vi "FR GUI DC meter setup.vi"(11 "DC meter":T2={"DC meter type"=enum."H/A/K 3458", "DC meter VISA"="", "NPLC"=10, "status ref"=refnum}) -> (3 "DC meter out":T2={"DC meter type"=enum."H/A/K 3458", "DC meter VISA"="", "NPLC"=10, "status ref"=refnum})   [LabVIEW 2020]
doc: "Use this template to build a producer/consumer design pattern with events to produce queue items. Use this design pattern instead of the User Interface Event Handler pattern for user interfaces when you want to execute code asynchronously in response to an event without slowing the user interface responsiveness."
uses:
  General DC meter/Type definitions/DC meter.ctl
  General DC meter/Type definitions/DC meter type.ctl
  <vilib>/Utility/error.llb/DialogType.ctl
  <vilib>/Utility/error.llb/Error Cluster From Error Code.vi
  <vilib>/ErrorRing/Error Ring.xnode
  external libraries/varilib/varilib.lvlib
panel:
  out "not tested label":string="This device is not\nyet fully tested!"
  in  "NPLC":i32=10 min=1
  in  "DC meter type":T1
  in  "VISA":refnum<visa-resource-name>
  out "gui_elements":refnum<vi>[](array[refnum])
  out "Status":string
  in  "save_and_quit":bool
  in  "test":bool
  in  "cancel":bool
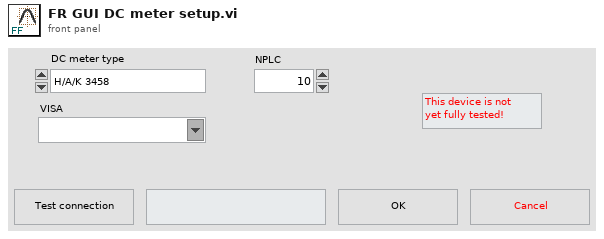
[diagram p1: front panel]
types:
  T1 = typedef "DC meter type.ctl" = enum16{"H/A/K 3458", "FLuke 8508A", "dummy"}
  T2 = typedef "DC meter.ctl" = cluster{"DC meter type":T1, "DC meter VISA":refnum<visa-resource-name>, "NPLC":i32, "status ref":refnum<vi>}
  T3 = typedef "DialogType.ctl" = u16
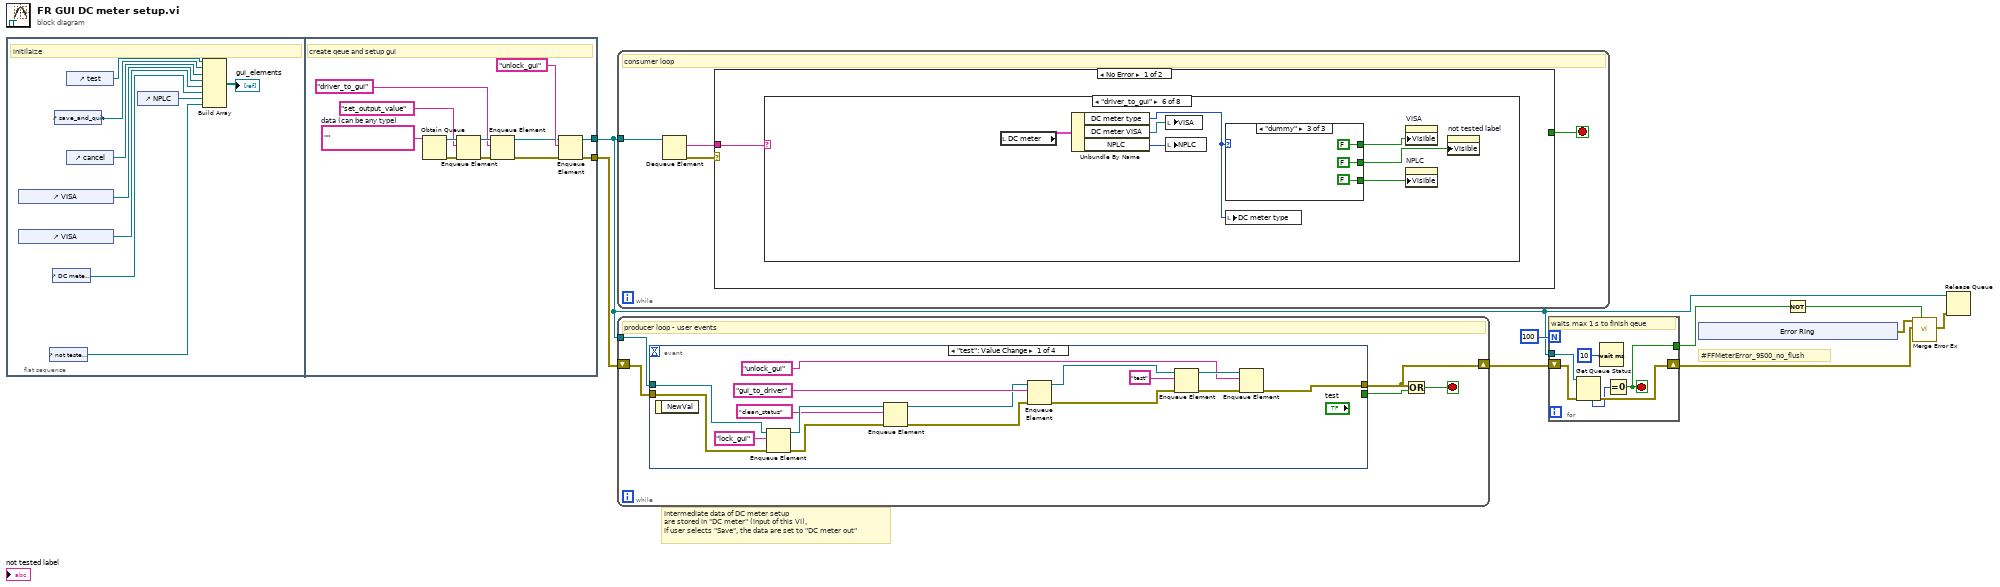
[diagram p0: block diagram]
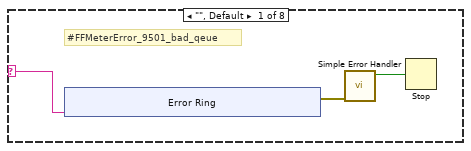
[diagram p2: hidden frame]
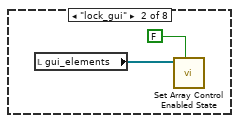
[diagram p3: hidden frame]
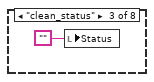
[diagram p4: hidden frame]
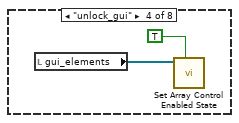
[diagram p5: hidden frame]
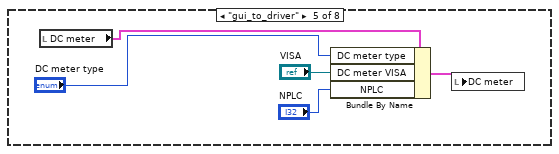
[diagram p6: hidden frame]
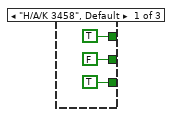
[diagram p7: hidden frame]
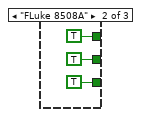
[diagram p8: hidden frame]
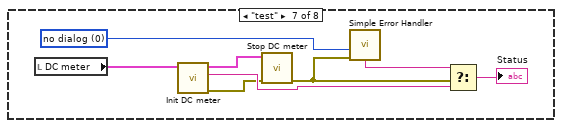
[diagram p9: hidden frame]
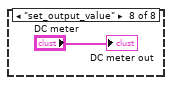
[diagram p10: hidden frame]
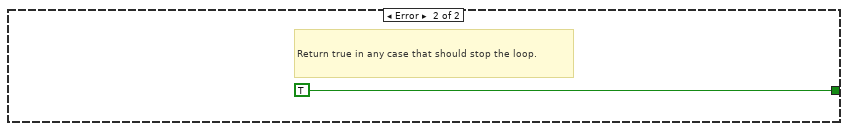
[diagram p11: hidden frame]
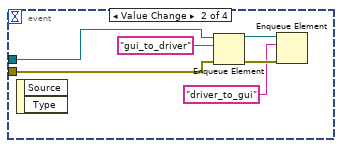
[diagram p12: hidden frame]
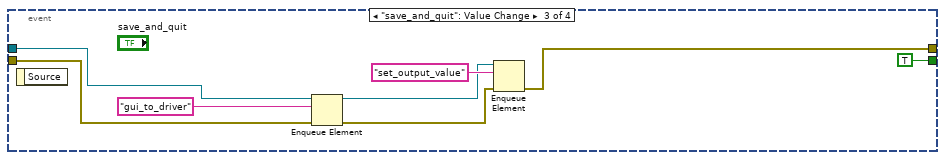
[diagram p13: hidden frame]
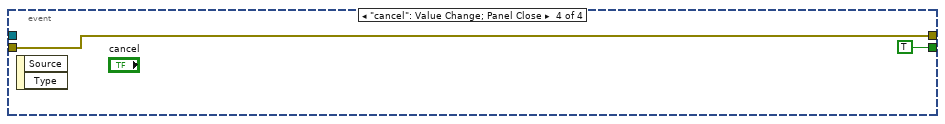
[diagram p14: hidden frame]
diagram:
  # "#FFMeterError_9500_no_flush"
  # "intermediate data of DC meter setup\nare stored in \"DC meter\" (input of this VI),\nif user selects \"Save\", the data are set to \"DC meter out\""
  n1 = flat-sequence {
    tunnel: [w23] -> w2
    tunnel: [w21] -> w1
    frame #0 {
      # "initilaize"
      n2 = control-ref of="VISA"() -> (w12:refnum<vi>)
      n3 = control-ref of="VISA"() -> (w14:refnum<vi>)
      n4 = control-ref of="not tested label"() -> (w10:refnum<vi>)
      n5 = control-ref of="DC meter type"() -> (w13:refnum<vi>)
      n6 = control-ref of="save_and_quit"() -> (w17:refnum<vi>)
      n7 = control-ref of="test"() -> (w18:refnum<vi>)
      n8 = control-ref of="cancel"() -> (w16:refnum<vi>)
      n9 = control-ref of="NPLC"() -> (w11:refnum<vi>)
      n10 = Build Array(w18, w17, w16, w12, w14, w13, w11, w10) -> (→"gui_elements":refnum<vi>[])
    }
    frame #1 {
      w22 = ""  # data (can be any type)
      # "create qeue and setup gui"
      n11 = Obtain Queue(element data type=w22) -> (queue out=w27:refnum<queue>, error out=w29:errorcluster)  [unwired: 4 in, 1 out]
      n12 = Enqueue Element(queue=w27, element="set_output_value", error in (no error)=w29) -> (queue out=w28:refnum<queue>, error out=w30:errorcluster)  [unwired: 1 in, 1 out]
      n13 = Enqueue Element(queue=w28, element="driver_to_gui", error in (no error)=w30) -> (queue out=w19:refnum<queue>, error out=w20:errorcluster)  [unwired: 1 in, 1 out]
      n14 = Enqueue Element(queue=w19, element="unlock_gui", error in (no error)=w20) -> (queue out=w23:refnum<queue>, error out=w21:errorcluster)  [unwired: 1 in, 1 out]
    }
  }
  n15 = while {
    tunnel: w2 -> [w34]
    stop <- w31 stop-if-true
    # "consumer loop"
    n16 = Dequeue Element(queue=w34) -> (element=w32:string, error out=w33:errorcluster)  [unwired: 2 in, 2 out]
    n17 = case shown="No Error" w33 {
      tunnel: w32 -> [w35 _]
      tunnel: [_ TRUE] -> w31
      frame No Error {
        n18 = case shown="\"driver_to_gui\"" w35 {
          selector: w35 -> [w36 _ _ _ _ _ _ _]
          frame "", Default {
            # "#FFMeterError_9501_bad_qeue"
            n19 = xnode "Error Ring"("parameter 0"=w36) -> ("error out"=w38:errorcluster)
            n20 = call <vilib>:"Simple Error Handler.vi"("error in (no error)"=w38) -> ("error?"=w37:bool)  [unwired: 4 in, 4 out]
            n21 = Stop(stop? (T)=w37) -> ()
          }
          frame "lock_gui" {
            n22 = local read "gui_elements"() -> (w47:refnum<vi>[])
            n23 = call "Set Array Control Enabled State.vi"("enabled (T)"=FALSE, "reference array in"=w47) -> ()  [unwired: 8 in, 2 out]
          }
          frame "clean_status" {
            n24 = local write "Status"("") -> ()
          }
          frame "unlock_gui" {
            n25 = local read "gui_elements"() -> (w50:refnum<vi>[])
            n26 = call "Set Array Control Enabled State.vi"("enabled (T)"=TRUE, "reference array in"=w50) -> ()  [unwired: 8 in, 2 out]
          }
          frame "gui_to_driver" {
            n27 = local read "DC meter"() -> (w54:T2)
            n28 = Bundle By Name(cluster=w54, "DC meter type"="DC meter type", "DC meter VISA"="VISA", "NPLC"="NPLC") -> (w55:T2)
            n29 = local write "DC meter"(w55) -> ()
          }
          frame "driver_to_gui" {
            n30 = local read "DC meter"() -> (w62:T2)
            n31 = Unbundle By Name(w62) -> ("DC meter type"=w59:T1, "DC meter VISA"=w61:refnum<visa-resource-name>, "NPLC"=w60:i32)
            n32 = local write "VISA"(w61) -> ()
            n33 = local write "NPLC"(w60) -> ()
            n34 = case shown="\"dummy\"" w59 {
              tunnel: [TRUE ("Visible") TRUE ("Visible") FALSE ("Visible")] -> w58
              tunnel: [TRUE ("Visible") TRUE ("Visible") FALSE ("Visible")] -> w57
              tunnel: [FALSE ("Visible") TRUE ("Visible") FALSE ("Visible")] -> w56
              frame "H/A/K 3458", Default {
              }
              frame "FLuke 8508A" {
              }
              frame "dummy" {
              }
            }
            n35 = local write "DC meter type"(w59) -> ()
            n36 = property on="VISA" class="VISAName"("Visible"=w57) -> ()  [unwired: 2 in, 2 out]
            n37 = property on="NPLC" class="DigNum (strict)"("Visible"=w58) -> ()  [unwired: 2 in, 2 out]
            n38 = property on="not tested label" class="Str"("Visible"=w56) -> ()  [unwired: 2 in, 2 out]
          }
          frame "test" {
            w79 = T3 0 items=["no dialog", "OK message", "continue or stop message", "OK message + warnings", "continue/stop + warnings"] ("type of dialog (OK msg:1)")
            n39 = local read "DC meter"() -> (w76:T2)
            n40 = call "Init DC meter.vi"("DC meter"=w76) -> ("error out"=w73:errorcluster, "Init status"=w75:string, "DC meter out"=w72:T2)  [unwired: 8 in]
            n41 = call "Stop DC meter.vi"("error in (no error)"=w73, "DC meter"=w72) -> ("error out"=w74:errorcluster)  [unwired: 8 in, 1 out]
            n42 = call <vilib>:"Simple Error Handler.vi"("type of dialog (OK msg:1)"=w79, "error in (no error)"=w74) -> ("message"=w78:string)  [unwired: 3 in, 4 out]
            n43 = Select(t=w78, s=w74, f=w75) -> (s? t:f=→"Status":string)
          }
          frame "set_output_value" {
            "DC meter out" <- "DC meter"
          }
        }
      }
      frame Error {
        # "Return true in any case that should stop the loop."
      }
    }
  }
  n44 = while {
    shift-right: [w82] -> w5
    shift-left: w1 -> [w85]
    tunnel: w2 -> [w86]
    stop <- w83 stop-if-true
    # "producer loop - user events"
    n45 = event shown="[0] \"test\": Value Change" {
      selector: _ -> [_ _ _ _]
      dyn-events: _ -> [_ _ _ _]
      timeout: _ -> [_ _ _ _]
      tunnel: w86 -> [w93 w107 w113 _]
      tunnel: w85 -> [w94 w108 w110 w118]
      tunnel: [w97 _ w109 w118] -> w82
      tunnel: [_ _ TRUE ("cancel") TRUE ("cancel")] -> w84
      event "test": Value Change {
        n46 = event-data() -> ()  [unwired: 1 in, 1 out]
        n47 = Enqueue Element(queue=w93, element="lock_gui", error in (no error)=w94) -> (queue out=w90:refnum<queue>, error out=w91:errorcluster)  [unwired: 1 in, 1 out]
        n48 = Enqueue Element(queue=w90, element="clean_status", error in (no error)=w91) -> (queue out=w88:refnum<queue>, error out=w89:errorcluster)  [unwired: 1 in, 1 out]
        n49 = Enqueue Element(queue=w88, element="gui_to_driver", error in (no error)=w89) -> (queue out=w100:refnum<queue>, error out=w101:errorcluster)  [unwired: 1 in, 1 out]
        n50 = Enqueue Element(queue=w100, element="test", error in (no error)=w101) -> (queue out=w96:refnum<queue>, error out=w98:errorcluster)  [unwired: 1 in, 1 out]
        n51 = Enqueue Element(queue=w96, element="unlock_gui", error in (no error)=w98) -> (error out=w97:errorcluster)  [unwired: 1 in, 2 out]
      }
      event Value Change {
        n52 = event-data() -> ()  [unwired: 1 in, 2 out]
        n53 = Enqueue Element(queue=w107, element="gui_to_driver", error in (no error)=w108) -> (queue out=w104:refnum<queue>, error out=w105:errorcluster)  [unwired: 1 in, 1 out]
        n54 = Enqueue Element(queue=w104, element="driver_to_gui", error in (no error)=w105) -> ()  [unwired: 1 in, 3 out]
      }
      event "save_and_quit": Value Change {
        n55 = event-data() -> ()  [unwired: 1 in, 1 out]
        n56 = Enqueue Element(queue=w113, element="gui_to_driver", error in (no error)=w110) -> (queue out=w112:refnum<queue>, error out=w111:errorcluster)  [unwired: 1 in, 1 out]
        n57 = Enqueue Element(queue=w112, element="set_output_value", error in (no error)=w111) -> (error out=w109:errorcluster)  [unwired: 1 in, 2 out]
      }
      event "cancel": Value Change; Panel Close {
        n58 = event-data() -> ()  [unwired: 1 in, 2 out]
      }
    }
    n59 = Or(x=w82, y=w84) -> (x .or. y?=w83:bool)
  }
  n60 = for {
    N: 100 -> [_]
    tunnel: w2 -> [w124]
    shift-right: [w122] -> w6
    shift-left: w5 -> [w123]
    tunnel: [w119] -> w3
    stop <- w119 stop-if-true
    # "waits max 1 s to finish qeue"
    n61 = Get Queue Status(queue=w124, error in (no error)=w123) -> (error out=w122:errorcluster, # elements in queue=w120:i32)  [unwired: 1 in, 6 out]
    n62 = Wait (ms)(milliseconds to wait=u32 10) -> ()  [unwired: 1 out]
    n63 = Equal To 0?(x=w120) -> (x = 0?=w119:bool)
  }
  n64 = xnode "Error Ring"() -> ("error out"=w7:errorcluster)
  n65 = Not(x=w3) -> (.not. x?=w8:bool)
  n66 = call "Merge Error Ex.vi"("Is error? (False)"=w8, "main error in (no error)"=w6, "second error in"=w7) -> ("error out"=w4:errorcluster)  [unwired: 8 in]
  n67 = Release Queue(queue=w2, error in (no error)=w4) -> ()  [unwired: 1 in, 3 out]
